vi "Add Version.vi"(8 "error in (no error)":errorcluster, 10 "Pkg Version":refnum<class "Package Version.lvclass">, 11 "Package in":refnum<class "Package.lvclass">) -> (0 "error out":errorcluster, 3 "Package out":refnum<class "Package.lvclass">)   [LabVIEW 2016, in "Packages.lvlib" / "Package.lvclass"]
uses:
  Package.lvclass
  Package Version_class/Package Version.lvclass
  Package.lvclass/Package.ctl
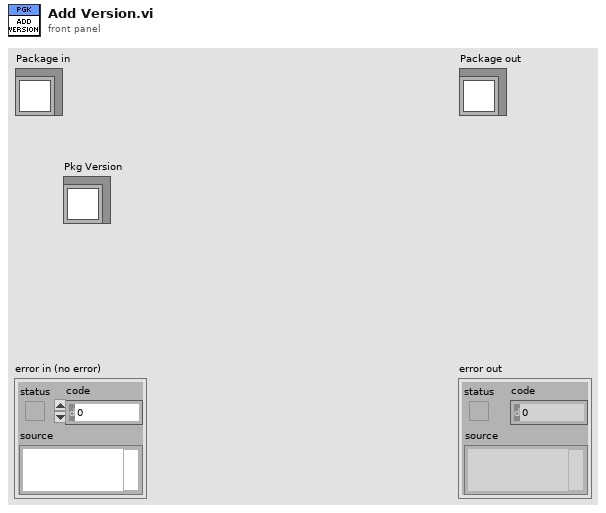
[diagram p1: front panel]
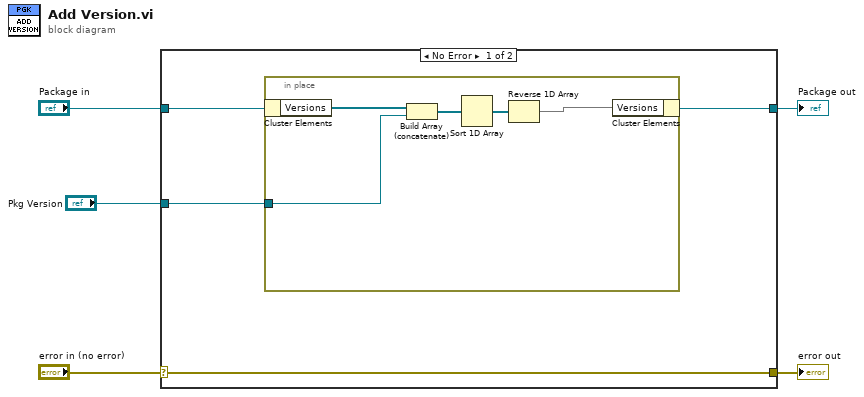
[diagram p0: block diagram]
diagram:
  n1 = case shown="No Error" "error in (no error)" {
    selector: "error in (no error)" -> [w9 w16]
    tunnel: [w9 w16] -> w4
    tunnel: [w7 w15] -> w2
    tunnel: "Package in" -> [w8 w15]
    tunnel: "Pkg Version" -> [w6 _]
    frame No Error {
      n2 = in-place {
        in-place-border: w6 -> [w10]
        n3 = in-place-cluster #1(w8) -> ("Versions"=w14:refnum<class "Package Version.lvclass">[])
        n4 = Build Array (concatenate)(w14, w10) -> (w13:refnum<class "Package Version.lvclass">[])
        n5 = Sort 1D Array(array=w13) -> (sorted array=w12:refnum<class "Package Version.lvclass">[])
        n6 = Reverse 1D Array(array=w12) -> (reversed array=w11:refnum<class "Package Version.lvclass">[])
        n7 = in-place-cluster #1("Versions"=w11) -> (w7:refnum<class "Package.lvclass">)
      }
    }
    frame Error {
    }
  }
  "error out" <- w4
  "Package out" <- w2
